vi "Setup.vi"(10 "Actor":refnum<class "Actor.lvclass">, 11 "Ex Event Actor in":refnum<class "Ex Event Actor.lvclass">) -> (3 "Ex Event Actor out":refnum<class "Ex Event Actor.lvclass">)   [LabVIEW 2021, in "Ex Event Actor.lvlib" / "Ex Event Actor.lvclass"]
uses:
  Ex Event Actor.lvclass
  Actor/Actor/Actor.lvclass
  Ex Event Actor.lvclass/Ex Event Actor.ctl
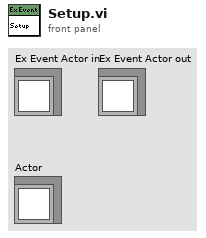
[diagram p1: front panel]
types:
  T1 = enum32{"Invalid", "Standard", "Closed", "Hidden", "Minimized", "Maximized"}
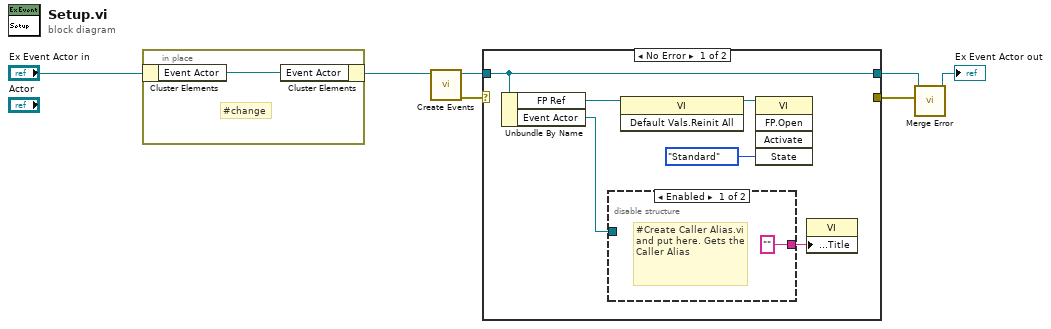
[diagram p0: block diagram]
diagram:
  n1 = in-place {
    # "#change"
    n2 = in-place-cluster #1("Ex Event Actor in") -> ("Event Actor"=w8:refnum<class "Event Actor.lvclass">)
    n3 = in-place-cluster #1("Event Actor"=w8) -> (w2:refnum<class "Ex Event Actor.lvclass">)
  }
  n4 = call "Create Events.vi"("Ex Event Actor in"=w2) -> ("error out"=w3:errorcluster, "Ex Event Actor out"=w4:refnum<class "Ex Event Actor.lvclass">)  [unwired: 9 in]
  n5 = case shown="No Error" w3 {
    selector: w3 -> [_ w16]
    tunnel: w4 -> [w9 w17]
    tunnel: [w9 w17] -> w7
    tunnel: [_ w16] -> w6
    frame No Error {
      n6 = Unbundle By Name(w9) -> ("FP Ref"=w12:refnum<vi>, "Event Actor"=w10:refnum<class "Event Actor.lvclass">)
      n7 = disable-structure shown="Enabled" {
        disable-tunnel: ["" ("Front Panel Window:Title") _] -> w11
        disable-tunnel: w10 -> [_ _]
        frame Enabled {
          # "#Create Caller Alias.vi\nand put here. Gets the Caller Alias"
        }
        frame Disabled {
        }
      }
      n8 = invoke class="VI" method="Default Vals.Reinit All"(reference=w12) -> (reference out=w13:refnum<vi>)  [unwired: 2 in, 2 out]
      n9 = invoke class="VI" method="FP.Open"(reference=w13, "State"=T1."Standard") -> ()  [unwired: 3 in, 5 out]
      n10 = property class="VI"("Front Panel.Title"=w11) -> ()  [unwired: 2 in, 2 out]
    }
    frame Error {
    }
  }
  n11 = call-dynamic "Merge Error.vi"("Error"=w6, "Ex Event Actor in"=w7) -> ("Ex Event Actor out"=→"Ex Event Actor out":refnum<class "Ex Event Actor.lvclass">)  [unwired: 9 in]
